vi "Sine.vi"(9 "phase(digree)":dbl=360.0 format="%#_13g", 10 "amplitude":dbl=220.0, 11 "frequency":dbl=50.0 format="%#_13g") -> (3 "data":sgl[](array[numeric]))   [LabVIEW 2020]
uses:
  <vilib>/measure/NI_MABase.lvlib
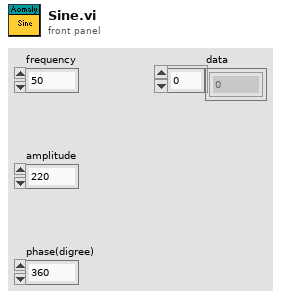
[diagram p1: front panel]
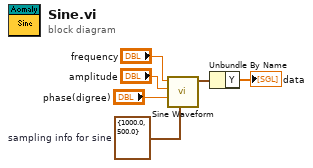
[diagram p0: block diagram]
diagram:
  w6 = cluster{"Fs":dbl, "#s":dbl} {"Fs"=1000.0, "#s"=500.0}  # sampling info for sine
  n1 = call <vilib>:"Sine Waveform.vi"("sampling info"=w6, "phase"="phase(digree)", "amplitude"="amplitude", "frequency"="frequency") -> ("signal out"=w3:waveform(dbl))  [unwired: 6 in, 1 out]
  n2 = Unbundle By Name(w3) -> ("Y"=→"data":dbl[])
